vi "CameraStatus.vi"() -> ()   [LabVIEW 2009]
panel:
  in  "camera status":string
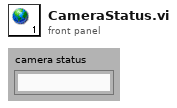
[diagram p1: front panel]
diagram:
